vi "setRoot.vi"(8 "error in (no error)":errorcluster, 10 "Root":refnum<data-value>, 11 "Graph in":refnum<class "Graph.lvclass">) -> (0 "error out":errorcluster, 3 "Graph out":refnum<class "Graph.lvclass">)   [LabVIEW 2009, in "Graph.lvclass"]
doc: "Sets the Root Node of the Graph."
uses:
  Graph.lvclass
  GraphNode/GraphNode.lvclass
  Graph.lvclass/Graph.ctl
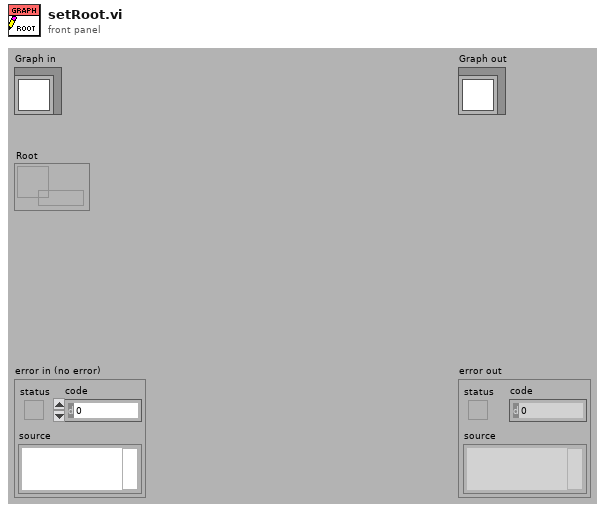
[diagram p1: front panel]
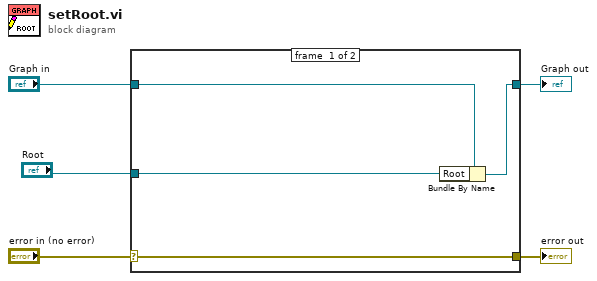
[diagram p0: block diagram]
diagram:
  n1 = case shown="No Error" "error in (no error)" {
    selector: "error in (no error)" -> [w9 w10]
    tunnel: [w9 w10] -> w4
    tunnel: [w7 w11] -> w2
    tunnel: "Graph in" -> [w8 w11]
    tunnel: "Root" -> [w6 _]
    frame #0 {
      n2 = Bundle By Name(cluster=w8, "Root"=w6) -> (w7:refnum<class "Graph.lvclass">)
    }
    frame #1 {
    }
  }
  "error out" <- w4
  "Graph out" <- w2
